vi "Hilbert Transform I18,1.vi"(0 "input":fxp<+/-,18,1>, 1 "reset":bool, 9 "input valid":bool) -> (4 "i":fxp<+/-,18,1>, 6 "q":fxp<+/-,37,3>, 10 "output valid":bool)   [LabVIEW 2018, in "NI PLL IP FPGA.lvlib"]
uses:
  NI PLL IP FPGA.lvlib
  <vilib>/rvi/IPIntegrationNode/IPINode_Typedef/niFpgaIPINodeSupportedFamilies.ctl
  <vilib>/rvi/IPIntegrationNode/IPINode_Utilities/niFpgaIPINodeSimCore.vi
  <vilib>/rvi/XilinxIP/XIPIN_XNode/niFpgaXIPIN.xnode
  hilbert/xsim.dir/hilbert_286C3DE52D9440B7A5661489EED6DA06/xsimk_286C3DE52D9440B7A5661489EED6DA06.dll
  <vilib>/rvi/IPIntegrationNode/IPINode_Xnode/niFpgaIPINode.xnode
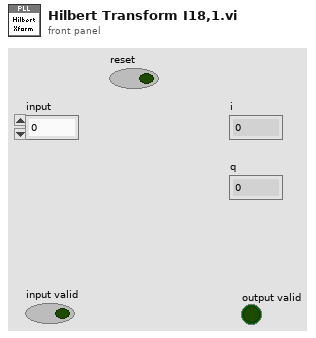
[diagram p1: front panel]
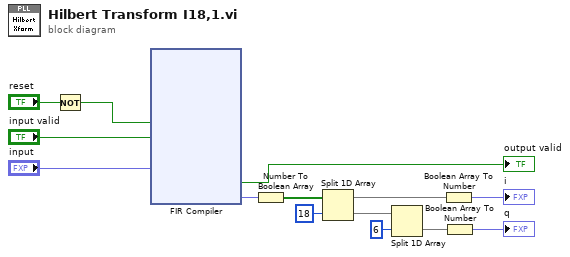
[diagram p0: block diagram]
diagram:
  n1 = Not(x="reset") -> (.not. x?=w1:bool)
  n2 = xnode ("FIR Compiler")("aresetn"=w1, "s_axis_data_tvalid"="input valid", "s_axis_data_tdata"="input") -> ("m_axis_data_tvalid"=→"output valid":bool, "m_axis_data_tdata"=w14:fxp<+,64,64>)  [unwired: 1 out]
  n3 = Number To Boolean Array(number=w14) -> (Boolean array=w13:bool[])
  n4 = Split 1D Array(array=w13, index=18) -> (first subarray=w11:bool[], second subarray=w10:bool[])
  n5 = Split 1D Array(array=w10, index=6) -> (second subarray=w8:bool[])  [unwired: 1 out]
  n6 = Boolean Array To Number(Boolean array=w11) -> (number=→"i":fxp<+/-,18,1>)
  n7 = Boolean Array To Number(Boolean array=w8) -> (number=→"q":fxp<+/-,37,3>)
